vi "quad_formula(SubVI).vi"(9 "c":dbl, 10 "b":dbl, 11 "a":dbl) -> (1 "String":string, 2 "Numeric":dbl, 3 "Numeric 2":dbl)   [LabVIEW 2026]
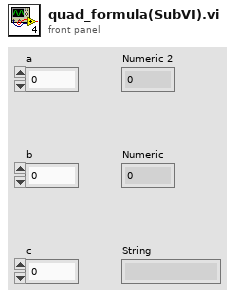
[diagram p1: front panel]
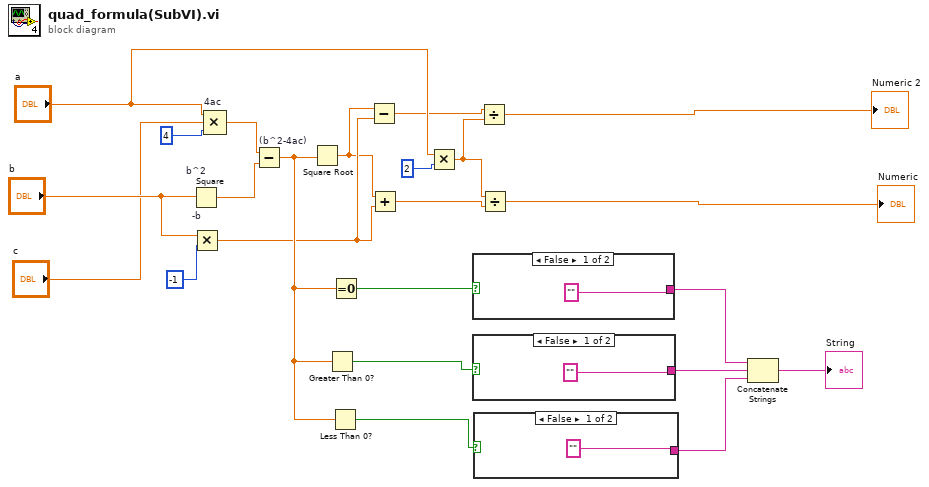
[diagram p0: block diagram]
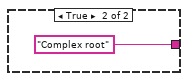
[diagram p2: hidden frame]
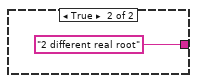
[diagram p3: hidden frame]
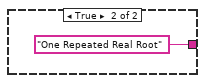
[diagram p4: hidden frame]
diagram:
  n1 = Square "b^2"(x="b") -> (x^2=w5:dbl)
  n2 = Multiply "-b"(x="b", y=-1) -> (x*y=w8:dbl)
  n3 = Compound Arithmetic op=MULTIPLY "4ac"("a", "c", 4) -> (w4:dbl)
  n4 = Subtract "(b^2-4ac)"(x=w4, y=w5) -> (x-y=w16:dbl)
  n5 = Square Root(x=w16) -> (sqrt(x)=w6:dbl)
  n6 = Greater Than 0?(x=w16) -> (x > 0?=w18:bool)
  n7 = Less Than 0?(x=w16) -> (x < 0?=w19:bool)
  n8 = Equal To 0?(x=w16) -> (x = 0?=w17:bool)
  n9 = Subtract(x=w6, y=w8) -> (x-y=w10:dbl)
  n10 = Add(x=w6, y=w8) -> (x+y=w11:dbl)
  n11 = Multiply(x="a", y=2) -> (x*y=w9:dbl)
  n12 = case shown="False" w17 {
    tunnel: ["" "One Repeated Real Root"] -> w20
    frame False {
    }
    frame True {
    }
  }
  n13 = case shown="False" w18 {
    tunnel: ["" "2 different real root"] -> w21
    frame False {
    }
    frame True {
    }
  }
  n14 = case shown="False" w19 {
    tunnel: ["" "Complex root"] -> w22
    frame False {
    }
    frame True {
    }
  }
  n15 = Divide(x=w10, y=w9) -> (x/y=→"Numeric 2":dbl)
  n16 = Divide(x=w9, y=w11) -> (x/y=→"Numeric":dbl)
  n17 = Concatenate Strings(w20, w21, w22) -> (→"String":string)
